vi "Run Acquisition.vi"(8 "error in (no error)":errorcluster, 11 "Channel in":refnum<class "Channel.lvclass">) -> (0 "error out":errorcluster, 3 "Channel out":refnum<class "Channel.lvclass">)   [LabVIEW 2018, in "Channel.lvclass"]
uses:
  Channel.lvclass
  State Machine/State Machine.lvclass/State Machine.ctl
  Channel.lvclass/Channel.ctl
  State Machine/State Machine.lvclass
  RxTx/RxTx.lvclass
  Interface/Interface.lvclass
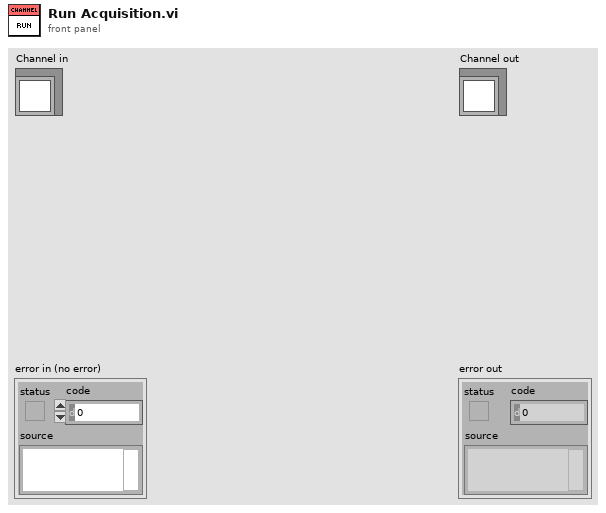
[diagram p1: front panel]
types:
  T1 = typedef "Shutter_mode typedef.ctl" = enum16{"Auto", "Open", "Close", "N/A (3)", "Open FVB Series", "Open Any Series"}
  T2 = typedef "ReadMode_mode typedef.ctl" = enum16{"Full Vertical Binning", "Multi-Track", "Random-Track", "Single-Track", "Image"}
  T3 = typedef "AcquisitionMode_mode typedef.ctl" = enum16{"Reserved (0)", "Single Scan", "Accumulate", "Kinetics", "Fast Kinetics", "Run Till Abort", "Reserved (6)", "Reserved (7)", "Reserved (8)", "Time Delayed Integration"}
  T4 = cluster{"EXPTIME":sgl, "PREAMP":enum16{"Gain 1", "Gain 2"}, "READOUT_RATE":enum16{"30 MHz", "20 MHz", "10 MHz", "1 MHz"}, "EM_GAIN":u16, "VBIN":u16, "INITIAL_LINE":u16, "INITIAL_COLUMN":u16, "FINAL_LINE":u16, "FINAL_COLUMN":u16, "#FRAMES":u32, "#CUBES":u32, "TRIGGER_MODE":enum16{"Internal", "External", "N/A", "N/A_1", "N/A_2", "N/A_3", "External Start"}, "HBIN":u16, "SHUTTER_TTL":enum16{"TTL Low", "TTL High"}, "SHUTTER_MODE":T1, "SHUTTER_OPENING_TIME":u16, "SHUTTER_CLOSING_TIME":u16, "VERTICAL_SHIFT_SPEED":u16, "READ_MODE":T2, "FRAME_TRANSFER":bool, "VERTICAL_CLOCK_VOLTAGE":enum16{"0", "+1", "+2", "+3", "+4"}, "ACQUISITION_MODE":T3, "AD_CHANNEL":u16, "EM_MODE":enum16{"Electron Multiplying", "Conventional"}}
  T5 = cluster{"CUBE_EXPOSURE_TIME":sgl, "CUBES_DONE":u16, "LAST_IMAGE_NAME":string, "DISK_SPACE":u16, "FRAMES_DONE":u16, "CCD_STATUS":string, "CURRENT_TEMPERATURE":i16, "TEMPERATURE_STATUS":string, "FRAME_EXPOSURE_TIME":u16, "CCD_ON_OFF":bool, "SERIAL_NUMBER":u16, "ACQUIRING":bool}
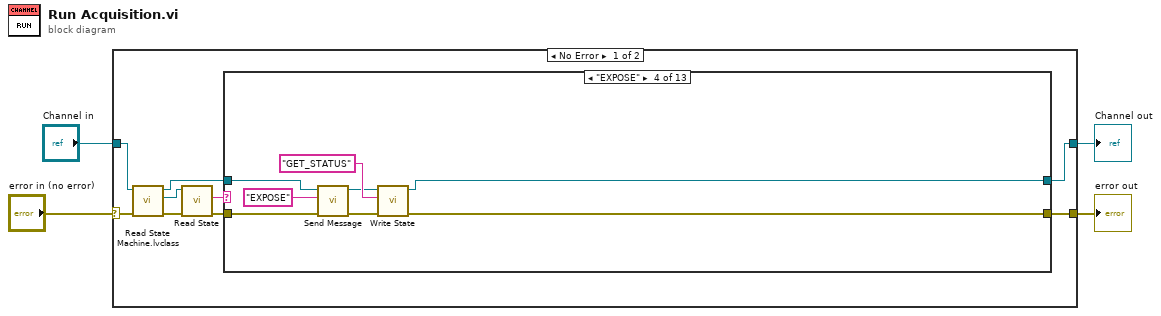
[diagram p0: block diagram]
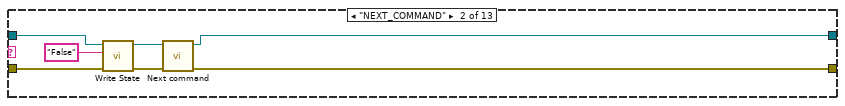
[diagram p3: hidden frame]
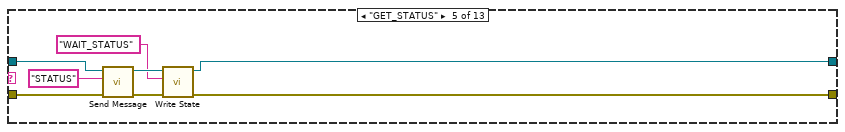
[diagram p5: hidden frame]
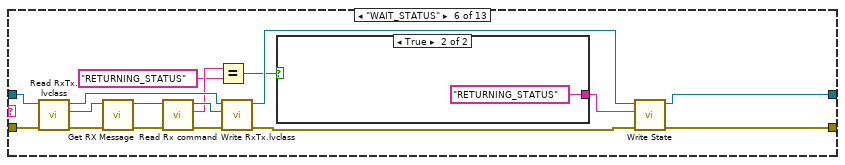
[diagram p6: hidden frame]
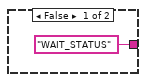
[diagram p7: hidden frame]
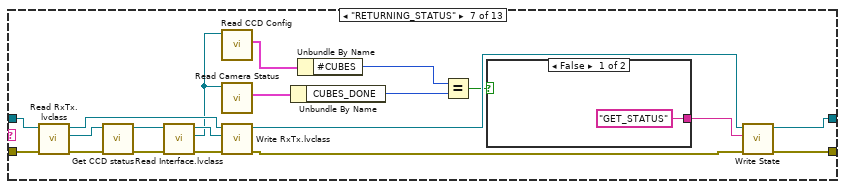
[diagram p8: hidden frame]
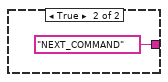
[diagram p9: hidden frame]
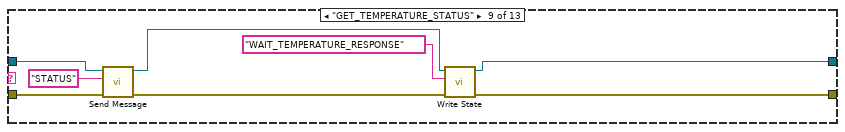
[diagram p11: hidden frame]
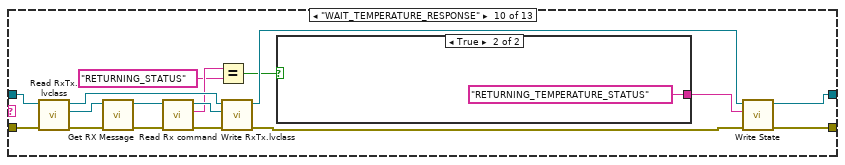
[diagram p12: hidden frame]
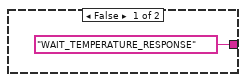
[diagram p13: hidden frame]
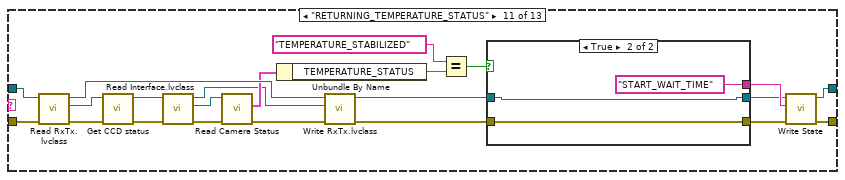
[diagram p14: hidden frame]
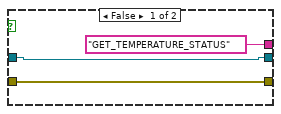
[diagram p15: hidden frame]
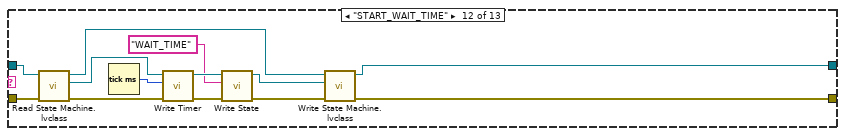
[diagram p16: hidden frame]
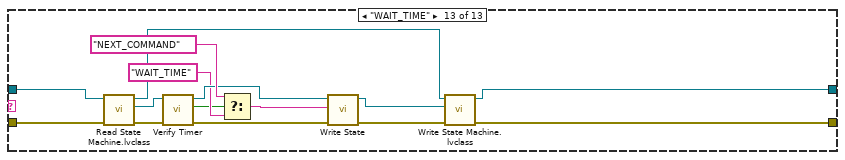
[diagram p17: hidden frame]
diagram:
  n1 = case shown="No Error" "error in (no error)" {
    selector: "error in (no error)" -> [w8 w168]
    tunnel: [w5 w168] -> w3
    tunnel: [w6 w167] -> w1
    tunnel: "Channel in" -> [w7 w167]
    frame No Error {
      n2 = call "Read State Machine.lvclass.vi"("error in (no error)"=w8, "Channel in"=w7) -> ("error out"=w12:errorcluster, "State Machine.lvclass"=w13:refnum<class "State Machine.lvclass">, "Channel out"=w10:refnum<class "Channel.lvclass">)  [unwired: 7 in]
      n3 = call-dynamic "Read State.vi"("error in (no error)"=w12, "State Machine in"=w13) -> ("error out"=w9:errorcluster, "State"=w11:string)  [unwired: 7 in, 1 out]
      n4 = case shown="\"EXPOSE\"" w11 {
        tunnel: w10 -> [w15 w21 w23 w32 w40 w57 w79 w83 w91 w95 w132 w151 w166]
        tunnel: w9 -> [w14 w22 w24 w29 w39 w56 w78 w82 w90 w96 w131 w150 w165]
        tunnel: [w15 w19 w23 w31 w35 w45 w75 w83 w86 w94 w128 w142 w162] -> w6
        tunnel: [w14 w18 w24 w30 w34 w46 w76 w82 w85 w93 w129 w143 w163] -> w5
        frame "False", Default {
        }
        frame "NEXT_COMMAND" {
          n5 = call "Write State.vi"("error in (no error)"=w22, "State"="False", "Channel in"=w21) -> ("error out"=w17:errorcluster, "Channel out"=w20:refnum<class "Channel.lvclass">)  [unwired: 7 in]
          n6 = call "Next command.vi"("error in (no error)"=w17, "Channel in"=w20) -> ("error out"=w18:errorcluster, "Channel out"=w19:refnum<class "Channel.lvclass">)  [unwired: 8 in]
        }
        frame "N/A2" {
        }
        frame "EXPOSE" {
          n7 = call "Send Message.vi"("error in (no error)"=w29, "message"="EXPOSE" ("State"), "Channel in"=w32) -> ("error out"=w26:errorcluster, "Channel out"=w27:refnum<class "Channel.lvclass">)  [unwired: 7 in]
          n8 = call "Write State.vi"("error in (no error)"=w26, "State"="GET_STATUS", "Channel in"=w27) -> ("error out"=w30:errorcluster, "Channel out"=w31:refnum<class "Channel.lvclass">)  [unwired: 7 in]
        }
        frame "GET_STATUS" {
          n9 = call "Send Message.vi"("error in (no error)"=w39, "message"="STATUS", "Channel in"=w40) -> ("error out"=w36:errorcluster, "Channel out"=w37:refnum<class "Channel.lvclass">)  [unwired: 7 in]
          n10 = call "Write State.vi"("error in (no error)"=w36, "State"="WAIT_STATUS" ("message"), "Channel in"=w37) -> ("error out"=w34:errorcluster, "Channel out"=w35:refnum<class "Channel.lvclass">)  [unwired: 7 in]
        }
        frame "WAIT_STATUS" {
          n11 = call "Read RxTx.lvclass.vi"("error in (no error)"=w56, "Channel in"=w57) -> ("error out"=w53:errorcluster, "RxTx.lvclass"=w52:refnum<class "RxTx.lvclass">, "Channel out"=w49:refnum<class "Channel.lvclass">)  [unwired: 7 in]
          n12 = call "Get RX Message.vi"("error in (no error)"=w53, "RxTx in"=w52) -> ("error out"=w54:errorcluster, "RxTx out"=w55:refnum<class "RxTx.lvclass">)  [unwired: 8 in]
          n13 = call "Read Rx command.vi"("error in (no error)"=w54, "RxTx in"=w55) -> ("error out"=w51:errorcluster, "Rx Command"=w42:string, "RxTx out"=w50:refnum<class "RxTx.lvclass">)  [unwired: 7 in]
          n14 = Equal?(x=w42, y="RETURNING_STATUS") -> (x = y?=w44:bool)
          n15 = call "Write RxTx.lvclass.vi"("error in (no error)"=w51, "RxTx.lvclass"=w50, "Channel in"=w49) -> ("error out"=w47:errorcluster, "Channel out"=w48:refnum<class "Channel.lvclass">)  [unwired: 7 in]
          n16 = case shown="True" w44 {
            tunnel: ["WAIT_STATUS" "RETURNING_STATUS"] -> w43
            frame False {
            }
            frame True {
            }
          }
          n17 = call "Write State.vi"("error in (no error)"=w47, "State"=w43, "Channel in"=w48) -> ("error out"=w46:errorcluster, "Channel out"=w45:refnum<class "Channel.lvclass">)  [unwired: 7 in]
        }
        frame "RETURNING_STATUS" {
          n18 = call "Read RxTx.lvclass.vi"("error in (no error)"=w78, "Channel in"=w79) -> ("error out"=w73:errorcluster, "RxTx.lvclass"=w74:refnum<class "RxTx.lvclass">, "Channel out"=w77:refnum<class "Channel.lvclass">)  [unwired: 7 in]
          n19 = call "Get CCD status.vi"("error in (no error)"=w73, "RxTx in"=w74) -> ("error out"=w61:errorcluster, "RxTx out"=w62:refnum<class "RxTx.lvclass">)  [unwired: 8 in]
          n20 = call "Read Interface.lvclass.vi"("error in (no error)"=w61, "RxTx in"=w62) -> ("error out"=w60:errorcluster, "Interface.lvclass"=w69:refnum<class "Interface.lvclass">, "RxTx out"=w70:refnum<class "RxTx.lvclass">)  [unwired: 7 in]
          n21 = call "Read CCD Config.vi"("Interface in"=w69) -> ("CCD Config"=w68:T4)  [unwired: 8 in, 2 out]
          n22 = call "Read Camera Status.vi"("Interface in"=w69) -> ("Camera Status"=w72:T5)  [unwired: 8 in, 2 out]
          n23 = call "Write RxTx.lvclass.vi"("error in (no error)"=w60, "RxTx.lvclass"=w70, "Channel in"=w77) -> ("error out"=w66:errorcluster, "Channel out"=w67:refnum<class "Channel.lvclass">)  [unwired: 7 in]
          n24 = Unbundle By Name(w72) -> ("CUBES_DONE"=w64:u16)
          n25 = Unbundle By Name(w68) -> ("#CUBES"=w65:u32)
          n26 = Equal?(x=w65, y=w64) -> (x = y?=w63:bool)
          n27 = case shown="False" w63 {
            tunnel: ["GET_STATUS" ("State") "NEXT_COMMAND" ("State")] -> w71
            frame False {
            }
            frame True {
            }
          }
          n28 = call "Write State.vi"("error in (no error)"=w66, "State"=w71, "Channel in"=w67) -> ("error out"=w76:errorcluster, "Channel out"=w75:refnum<class "Channel.lvclass">)  [unwired: 7 in]
        }
        frame "N/A" {
        }
        frame "GET_TEMPERATURE_STATUS" {
          n29 = call "Send Message.vi"("error in (no error)"=w90, "message"="STATUS", "Channel in"=w91) -> ("error out"=w87:errorcluster, "Channel out"=w88:refnum<class "Channel.lvclass">)  [unwired: 7 in]
          n30 = call "Write State.vi"("error in (no error)"=w87, "State"="WAIT_TEMPERATURE_RESPONSE" ("message"), "Channel in"=w88) -> ("error out"=w85:errorcluster, "Channel out"=w86:refnum<class "Channel.lvclass">)  [unwired: 7 in]
        }
        frame "WAIT_TEMPERATURE_RESPONSE" {
          n31 = call "Read RxTx.lvclass.vi"("error in (no error)"=w96, "Channel in"=w95) -> ("error out"=w106:errorcluster, "RxTx.lvclass"=w105:refnum<class "RxTx.lvclass">, "Channel out"=w102:refnum<class "Channel.lvclass">)  [unwired: 7 in]
          n32 = call "Get RX Message.vi"("error in (no error)"=w106, "RxTx in"=w105) -> ("error out"=w107:errorcluster, "RxTx out"=w108:refnum<class "RxTx.lvclass">)  [unwired: 8 in]
          n33 = call "Read Rx command.vi"("error in (no error)"=w107, "RxTx in"=w108) -> ("error out"=w104:errorcluster, "Rx Command"=w97:string, "RxTx out"=w103:refnum<class "RxTx.lvclass">)  [unwired: 7 in]
          n34 = Equal?(x=w97, y="RETURNING_STATUS") -> (x = y?=w99:bool)
          n35 = call "Write RxTx.lvclass.vi"("error in (no error)"=w104, "RxTx.lvclass"=w103, "Channel in"=w102) -> ("error out"=w100:errorcluster, "Channel out"=w101:refnum<class "Channel.lvclass">)  [unwired: 7 in]
          n36 = case shown="True" w99 {
            tunnel: ["WAIT_TEMPERATURE_RESPONSE" "RETURNING_TEMPERATURE_STATUS"] -> w98
            frame False {
            }
            frame True {
            }
          }
          n37 = call "Write State.vi"("error in (no error)"=w100, "State"=w98, "Channel in"=w101) -> ("error out"=w93:errorcluster, "Channel out"=w94:refnum<class "Channel.lvclass">)  [unwired: 7 in]
        }
        frame "RETURNING_TEMPERATURE_STATUS" {
          n38 = call "Read RxTx.lvclass.vi"("error in (no error)"=w131, "Channel in"=w132) -> ("error out"=w126:errorcluster, "RxTx.lvclass"=w127:refnum<class "RxTx.lvclass">, "Channel out"=w130:refnum<class "Channel.lvclass">)  [unwired: 7 in]
          n39 = call "Get CCD status.vi"("error in (no error)"=w126, "RxTx in"=w127) -> ("error out"=w124:errorcluster, "RxTx out"=w125:refnum<class "RxTx.lvclass">)  [unwired: 8 in]
          n40 = call "Read Interface.lvclass.vi"("error in (no error)"=w124, "RxTx in"=w125) -> ("error out"=w122:errorcluster, "Interface.lvclass"=w123:refnum<class "Interface.lvclass">, "RxTx out"=w115:refnum<class "RxTx.lvclass">)  [unwired: 7 in]
          n41 = call "Read Camera Status.vi"("error in (no error)"=w122, "Interface in"=w123) -> ("error out"=w116:errorcluster, "Camera Status"=w121:T5)  [unwired: 7 in, 1 out]
          n42 = Unbundle By Name(w121) -> ("TEMPERATURE_STATUS"=w120:string)
          n43 = call "Write RxTx.lvclass.vi"("error in (no error)"=w116, "RxTx.lvclass"=w115, "Channel in"=w130) -> ("error out"=w114:errorcluster, "Channel out"=w112:refnum<class "Channel.lvclass">)  [unwired: 7 in]
          n44 = Equal?(x="TEMPERATURE_STABILIZED" ("State"), y=w120) -> (x = y?=w118:bool)
          n45 = case shown="True" w118 {
            tunnel: ["GET_TEMPERATURE_STATUS" ("State") "START_WAIT_TIME" ("State")] -> w117
            tunnel: w114 -> [w134 w136]
            tunnel: [w134 w136] -> w113
            tunnel: w112 -> [w133 w137]
            tunnel: [w133 w137] -> w111
            frame False {
            }
            frame True {
            }
          }
          n46 = call "Write State.vi"("error in (no error)"=w113, "State"=w117, "Channel in"=w111) -> ("error out"=w129:errorcluster, "Channel out"=w128:refnum<class "Channel.lvclass">)  [unwired: 7 in]
        }
        frame "START_WAIT_TIME" {
          n47 = call "Read State Machine.lvclass.vi"("error in (no error)"=w150, "Channel in"=w151) -> ("error out"=w148:errorcluster, "State Machine.lvclass"=w149:refnum<class "State Machine.lvclass">, "Channel out"=w144:refnum<class "Channel.lvclass">)  [unwired: 7 in]
          n48 = Tick Count (ms)() -> (millisecond timer value=w145:u32)
          n49 = call "Write Timer.vi"("error in (no error)"=w148, "Timer"=w145, "State Machine in"=w149) -> ("error out"=w146:errorcluster, "State Machine out"=w147:refnum<class "State Machine.lvclass">)  [unwired: 7 in]
          n50 = call-dynamic "Write State.vi"("error in (no error)"=w146, "State"="WAIT_TIME", "State Machine in"=w147) -> ("error out"=w140:errorcluster, "State Machine out"=w141:refnum<class "State Machine.lvclass">)  [unwired: 7 in]
          n51 = call "Write State Machine.lvclass.vi"("error in (no error)"=w140, "State Machine.lvclass"=w141, "Channel in"=w144) -> ("error out"=w143:errorcluster, "Channel out"=w142:refnum<class "Channel.lvclass">)  [unwired: 7 in]
        }
        frame "WAIT_TIME" {
          n52 = call "Read State Machine.lvclass.vi"("error in (no error)"=w165, "Channel in"=w166) -> ("error out"=w158:errorcluster, "State Machine.lvclass"=w159:refnum<class "State Machine.lvclass">, "Channel out"=w164:refnum<class "Channel.lvclass">)  [unwired: 7 in]
          n53 = call "Verify Timer.vi"("error in (no error)"=w158, "State Machine in"=w159) -> ("error out"=w154:errorcluster, "Time out"=w152:bool, "State Machine out"=w155:refnum<class "State Machine.lvclass">)  [unwired: 6 in, 1 out]
          n54 = Select(t="NEXT_COMMAND", s=w152, f="WAIT_TIME") -> (s? t:f=w156:string)
          n55 = call-dynamic "Write State.vi"("error in (no error)"=w154, "State"=w156, "State Machine in"=w155) -> ("error out"=w160:errorcluster, "State Machine out"=w161:refnum<class "State Machine.lvclass">)  [unwired: 7 in]
          n56 = call "Write State Machine.lvclass.vi"("error in (no error)"=w160, "State Machine.lvclass"=w161, "Channel in"=w164) -> ("error out"=w163:errorcluster, "Channel out"=w162:refnum<class "Channel.lvclass">)  [unwired: 7 in]
        }
      }
    }
    frame Error {
    }
  }
  "error out" <- w3
  "Channel out" <- w1
